vi "calibration value.vi"(1 "Caibration Date":u16(ring) items=["first calibration - 7/31", "7/31-current"]) -> (0 "Numeric":i32)   [LabVIEW 2017]
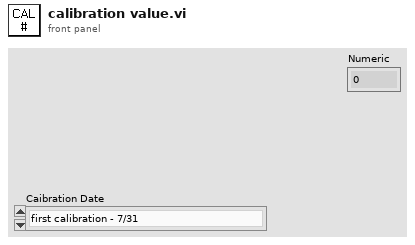
[diagram p1: front panel]
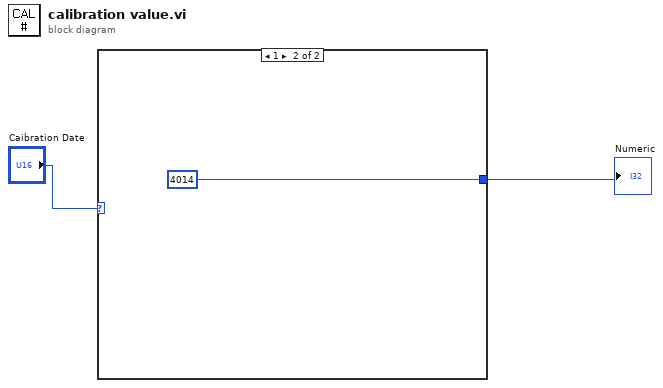
[diagram p0: block diagram]
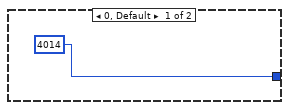
[diagram p2: hidden frame]
diagram:
  n1 = case shown="1" "Caibration Date" {
    tunnel: [4014 4014] -> w1
    frame 0, Default {
    }
    frame 1 {
    }
  }
  "Numeric" <- w1
